vi "Load Maze Gen.vi"(8 "error in (no error)":errorcluster, 11 "Maze Level":T1) -> (0 "error out":errorcluster, 3 "MazeGen":refnum<class "MazeGen.lvclass">)   [LabVIEW 2020, in "Maze.lvlib" / "MazeGen.lvclass"]
doc: "Loads the PPL that contains the logic for generating the specific maze level. <b>Basic</b> is built into the MazeGen class but other algorithms are loaded dynamically from disk to support being distributed after the start of the challenge.\n\n<b>Errors</b>\n\n<b>-124100</b> is thrown if the specific algorithm (PPL) was not found or able to be loaded."
uses:
  MazeGen.lvclass
  Maze Level.ctl
  <vilib>/Utility/LVLibp/NI_PackedLibraryUtility.lvlib
  Maze.lvlib
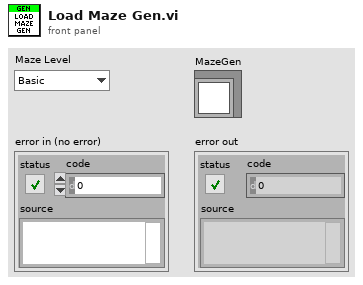
[diagram p1: front panel]
types:
  T1 = typedef "Maze.lvlib/Maze Level.ctl" = enum16{"Basic", "Intermediate", "Advanced", "Quantum"}
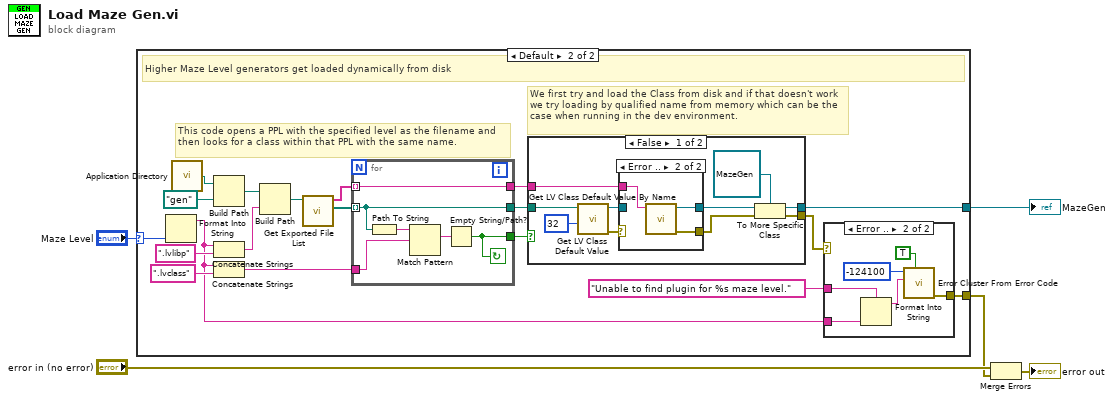
[diagram p0: block diagram]
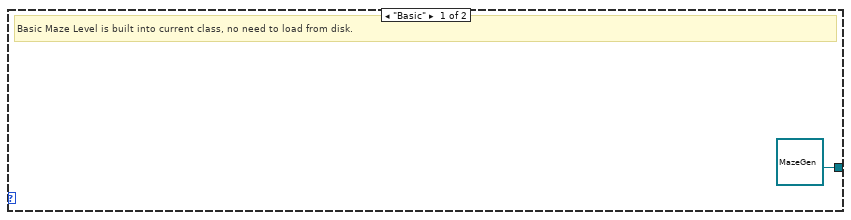
[diagram p2: hidden frame]
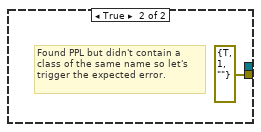
[diagram p5: hidden frame]
diagram:
  n1 = case shown="Default" "Maze Level" {
    selector: "Maze Level" -> [_ w25]
    tunnel: [refnum<class "MazeGen.lvclass"> refnum ("Maze.lvlib:MazeGen.lvclass") w11] -> w4
    tunnel: [_ w8] -> w1
    frame "Basic" {
      # "Basic Maze Level is built into current class, no need to load from disk."
    }
    frame Default {
      # "We first try and load the Class from disk and if that doesn't work we try loading by qualified name from memory which can be the case when running in the dev environment."
      # "This code opens a PPL with the specified level as the filename and then looks for a class within that PPL with the same name."
      # "Higher Maze Level generators get loaded dynamically from disk"
      n2 = Format Into String(w25) -> (resulting string=w7:string)  [unwired: 3 in, 1 out]
      n3 = call <vilib>:"Application Directory.vi"() -> ("Application Directory"=w23:path)
      n4 = Build Path(base path=w23, name or relative path=path "gen") -> (appended path=w21:path)
      n5 = Concatenate Strings(w7, ".lvlibp" ("string")) -> (w19:string)
      n6 = Concatenate Strings(w7, ".lvclass" ("string")) -> (w16:string)
      n7 = Build Path(base path=w21, name or relative path=w19) -> (appended path=w18:path)
      n8 = call <vilib>:"Get Exported File List.vi"("packed library path"=w18) -> ("paths"=w17:path[], "qualified names"=w13:string[])  [unwired: 8 in, 1 out]
      n9 = for {
        tunnel: w17 -> [w52] mode=indexing
        tunnel: [w52] -> w14
        tunnel: w16 -> [w50]
        tunnel: [w48] -> w15
        tunnel: w13 -> [w47] mode=indexing
        tunnel: [w47] -> w12
        stop <- w48 continue-if-true
        n10 = Path To String(path=w52) -> (string=w51:string)
        n11 = Match Pattern(string=w51, regular expression=w50) -> (match substring=w49:string)  [unwired: 1 in, 3 out]
        n12 = Empty String/Path?(string/path=w49) -> (empty?=w48:bool)
      }
      n13 = case shown="False" w15 {
        tunnel: w14 -> [w41 _]
        tunnel: w12 -> [w38 _]
        tunnel: [w34 _] -> w11
        tunnel: [w32 errorcluster {"status"=TRUE, "code"=1, "source"=""} ("error out")] -> w9
        frame False {
          n14 = call <vilib>:"Get LV Class Default Value.vi"("options"=u32 32, "class path"=w41) -> ("error out"=w39:errorcluster, "object"=w37:refnum<class>)  [unwired: 8 in]
          n15 = case shown="Error .." w39 {
            tunnel: w38 -> [_ w45]
            tunnel: w37 -> [w42 _]
            tunnel: [w42 w44] -> w36
            tunnel: [_ w43] -> w33
            frame No Error {
            }
            frame Error {
              n16 = call <vilib>:"Get LV Class Default Value By Name.vi"("class name"=w45) -> ("error out"=w43:errorcluster, "object"=w44:refnum<class>)  [unwired: 9 in]
            }
          }
          n17 = To More Specific Class(target class=refnum<class "MazeGen.lvclass"> refnum ("Maze.lvlib:MazeGen.lvclass"), reference=w36, error in=w33) -> (specific class reference=w34:refnum<class "MazeGen.lvclass">, error out=w32:errorcluster)
        }
        frame True {
          # "Found PPL but didn't contain a class of the same name so let's trigger the expected error."
        }
      }
      n18 = case shown="Error .." w9 {
        tunnel: "Unable to find plugin for %s maze level." -> [_ w28]
        tunnel: [_ w27] -> w8
        tunnel: w7 -> [_ w26]
        frame No Error {
        }
        frame Error {
          n19 = Format Into String(format string=w28, w26) -> (resulting string=w31:string)  [unwired: 2 in, 1 out]
          n20 = call <vilib>:"Error Cluster From Error Code.vi"("show call chain? (False)"=TRUE, "error message (\"\")"=w31, "error code (0)"=-124100) -> ("error out"=w27:errorcluster)  [unwired: 6 in]
        }
      }
    }
  }
  "MazeGen" <- w4
  n21 = Merge Errors("error in (no error)", w1) -> (→"error out":errorcluster)
